vi "Get Cell.vi"(0 "Display State In":T1, 5 "Row":i32, 7 "Column":i32, 9 "Container State":T6, 11 "error in (no error)":errorcluster) -> (4 "Display State Out":T1, 6 "String":string, 15 "error out":errorcluster)   [LabVIEW 2020, in "KTable.xctl"]
uses:
  KTable.xctl
  <vilib>/_xctls/Container State.ctl
  State.ctl
  ColumnSpec.ctl
  ColumnType.ctl
  Table Properties.ctl
  Events.ctl
  Event Data.ctl
  Event Type.ctl
  Array Manipulation VIs/Array-Dimensions (2D string).vi
  <vilib>/_xctls/XControlSupport.lvlib
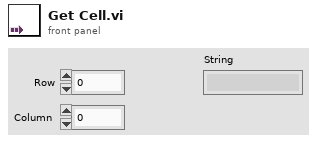
[diagram p1: front panel]
types:
  T1 = typedef "KTable.xctl/State.ctl" = cluster{"Columns":T2[], "Listbox":refnum<vi>, "Default row":string[], "Properties":T4, "Events":T5, "Locked":bool[][], "Size":cluster{"Rows":i32, "Columns":i32}, "rings":i32[][], "DefColors":u32[]}
  T2 = typedef "KTable.xctl/ColumnSpec.ctl" = cluster{"Name":string, "Type":T3, "Width":i32, "Strings":string[], "Position":enum16{"Left", "Center", "Right"}, "locked":bool, "cds":cluster{"Strings":string[]}[][], "Hide NaN":bool}
  T3 = typedef "KTable.xctl/ColumnType.ctl" = enum16{"String", "Enum", "Int", "Double", "Boolean", "Ring", "Formula", "Color"}
  T4 = typedef "KTable.xctl/Table Properties.ctl" = cluster{"Vertical scrollbar":bool, "User add/delete":bool, "Max rows":i32, "Row headers":bool}
  T5 = typedef "KTable.xctl/Events.ctl" = cluster{"Items Changed":refnum<user-event>}
  T6 = typedef "XControlSupport.lvlib/Container State.ctl" = cluster{"Indicator?":bool, "Run Mode?":bool, " Refnum":refnum<vi>}
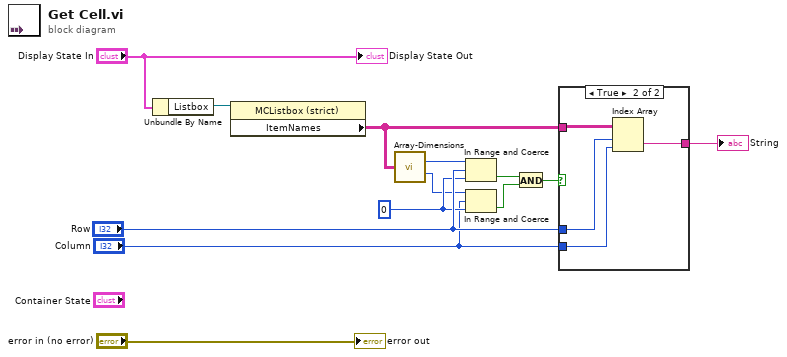
[diagram p0: block diagram]
diagram:
  w4 = 0
  n1 = Unbundle By Name("Display State In") -> ("Listbox"=w11:refnum<vi>)
  n2 = property class="MCListbox (strict)"(reference=w11) -> ("ItemNames"=w10:string[][])  [unwired: 1 in, 2 out]
  n3 = call-poly "Array-Dimensions.vi"("2D Array"=w10) -> ("# rows"=w8:i32, "# columns"=w3:i32)  [unwired: 13 in]
  n4 = In Range and Coerce(upper limit=w8, x="Row", lower limit=w4) -> (In Range?=w5:bool)  [unwired: 1 out]
  n5 = In Range and Coerce(upper limit=w3, x="Column", lower limit=w4) -> (In Range?=w1:bool)  [unwired: 1 out]
  n6 = And(x=w5, y=w1) -> (x .and. y?=w6:bool)
  n7 = case shown="True" w6 {
    tunnel: w10 -> [_ w17]
    tunnel: "Row" -> [_ w16]
    tunnel: "Column" -> [_ w15]
    tunnel: [_ w14] -> w9
    frame False {
    }
    frame True {
      n8 = Index Array(array=w17, index (row)=w16, index (col)=w15) -> (element=w14:string)
    }
  }
  "String" <- w9
  "Display State Out" <- "Display State In"
  "error out" <- "error in (no error)"
